vi "KE622x -- DCon Mode Set Stop Level.vi"(0 "Resource In":refnum<visa-resource-name>, 1 "Check For SCPI Errors? (T)":bool=TRUE, 7 "Stop Level In (A)":T1=0.001 min=-0.105 max=0.105 format="%.3p", 11 "error in (no error)":errorcluster, 12 "Read Back Set Value? (T)":bool=TRUE) -> (4 "Resource Out (dupl)":refnum<visa-resource-name>, 8 "Stop Level Out (A)":T1=0.001 min=-0.105 max=0.105 format="%.3p", 15 "error out":errorcluster)   [LabVIEW 2019, in "Keithley 622x.lvlib"]
uses:
  Keithley 622x.lvlib
  Typedefs/KE622x -- DCon Mode Start Stop Level.ctl
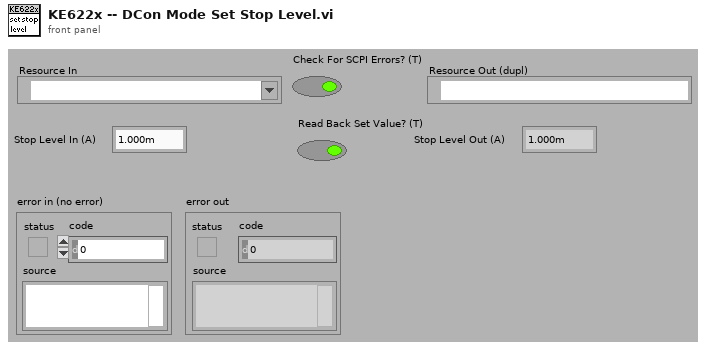
[diagram p1: front panel]
types:
  T1 = typedef "Keithley 622x.lvlib/KE622x -- DCon Mode Start Stop Level.ctl" = dbl
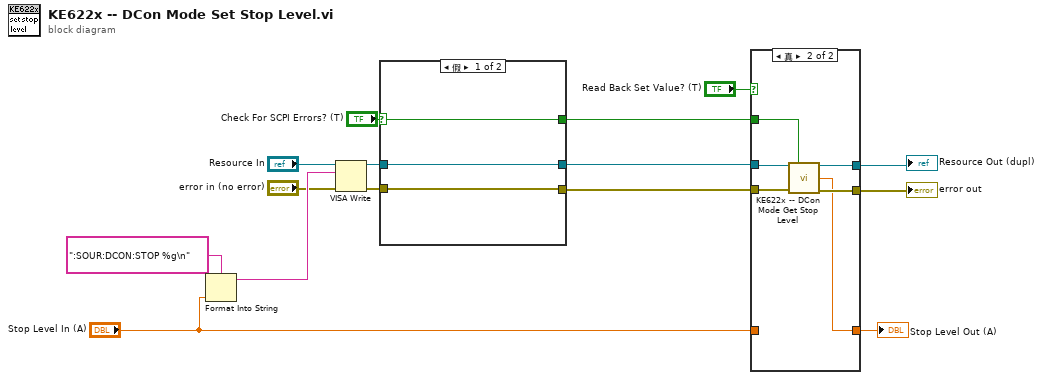
[diagram p0: block diagram]
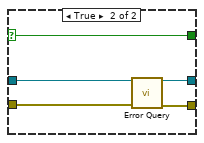
[diagram p3: hidden frame]
diagram:
  n1 = Format Into String(format string=":SOUR:DCON:STOP %g\n", "Stop Level In (A)") -> (resulting string=w13:string)  [unwired: 2 in, 1 out]
  n2 = VISA Write(VISA resource name="Resource In", write buffer=w13, error in (no error)="error in (no error)") -> (VISA resource name out=w10:refnum<visa-resource-name>, error out=w9:errorcluster)  [unwired: 1 out]
  n3 = case shown="假" "Check For SCPI Errors? (T)" {
    selector: "Check For SCPI Errors? (T)" -> [w16 w19]
    tunnel: w10 -> [w18 w23]
    tunnel: w9 -> [w17 w22]
    tunnel: [w17 w21] -> w6
    tunnel: [w18 w20] -> w7
    tunnel: [w16 w19] -> w5
    frame False {
    }
    frame True {
      n4 = call "Error Query.vi"("VISA Resource In"=w23, "error in (no error)"=w22) -> ("VISA Resource Out (dupl)"=w20:refnum<visa-resource-name>, "error out"=w21:errorcluster)  [unwired: 10 in, 2 out]
    }
  }
  n5 = case shown="真" "Read Back Set Value? (T)" {
    tunnel: w7 -> [w25 w32]
    tunnel: w6 -> [w24 w31]
    tunnel: w5 -> [_ w30]
    tunnel: [w25 w29] -> w4
    tunnel: [w24 w28] -> w3
    tunnel: "Stop Level In (A)" -> [w26 _]
    tunnel: [w26 w27] -> w1
    frame False {
    }
    frame True {
      n6 = call "KE622x -- DCon Mode Get Stop Level.vi"("Resource In"=w32, "Check For SCPI Errors? (T)"=w30, "error in (no error)"=w31) -> ("Resource Out (dupl)"=w29:refnum<visa-resource-name>, "Stop Level (A)"=w27:T1, "error out"=w28:errorcluster)  [unwired: 10 in]
    }
  }
  "Resource Out (dupl)" <- w4
  "error out" <- w3
  "Stop Level Out (A)" <- w1
